vi "Detect Cross Time.vi"(7 "CHn.Voltage":dbl[](array[numeric]), 9 "level":dbl=1.0) -> (8 "Crossing Time":dbl, 15 "error out":errorcluster)   [LabVIEW 2010]
uses:
  <vilib>/measure/mamon.llb/Trigger Detection for 1 Channel.vi
  <vilib>/measure/NI_MAPro.lvlib
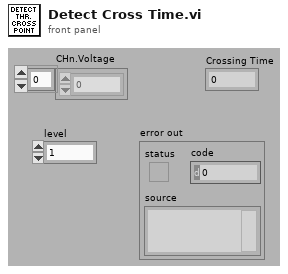
[diagram p1: front panel]
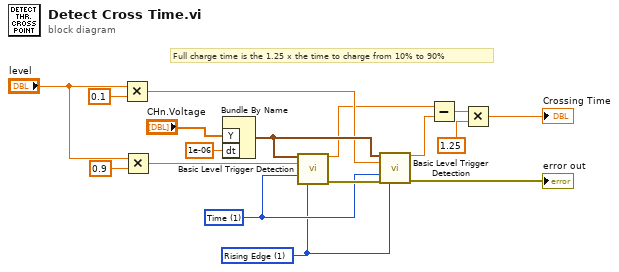
[diagram p0: block diagram]
diagram:
  w6 = u16 1 items=["Falling Edge", "Rising Edge"] ("trigger slope")
  w7 = u16 1 items=["Index", "Time"] ("location mode")
  # "Full charge time is the 1.25 x the time to charge from 10% to 90%"
  n1 = Multiply(x="level", y=0.1) -> (x*y=w8:dbl)
  n2 = Multiply(x="level", y=0.9) -> (x*y=w13:dbl)
  n3 = Bundle By Name("Y"="CHn.Voltage", "dt"=1e-06) -> (w11:waveform(dbl))  [unwired: 1 in]
  n4 = call-poly <vilib>:"Basic Level Trigger Detection.vi"("signal in"=w11, "level"=w13, "location mode"=w7, "trigger slope"=w6) -> ("trigger location"=w5:dbl, "error out"=w15:errorcluster)  [unwired: 9 in, 1 out]
  n5 = call-poly <vilib>:"Basic Level Trigger Detection.vi"("signal in"=w11, "level"=w8, "location mode"=w7, "error in (no error)"=w15, "trigger slope"=w6) -> ("trigger location"=w4:dbl, "error out"=→"error out":errorcluster)  [unwired: 8 in, 1 out]
  n6 = Subtract(x=w5, y=w4) -> (x-y=w3:dbl)
  n7 = Multiply(x=w3, y=1.25) -> (x*y=→"Crossing Time":dbl)
